vi "2.0 EMGtoOMG OFFLINE functional keyboard.vi"() -> ()   [LabVIEW 2018]
panel:
  out "charSearch":dbl[](array[numeric])
  in  "Sig 3":bool
  in  "Sig 2":bool
  in  "Sig 1":bool
  out "return value":string
  out "Array":string[](array[string])
  out "c":i32[](array[numeric])
  out "state":dbl[](array[numeric])
  out "charSearch":dbl[](array[numeric])
  out "seq70-104":dbl[](array[numeric])
  out "seq00-34":dbl[](array[numeric])
  out "setID":dbl[](array[numeric])
  out "seq35-69":dbl[](array[numeric])
  in  "Amplitude 3":dbl=1.0 caption="Amplitude"
  in  "Amplitude 2":dbl=1.0 caption="Amplitude"
  in  "Amplitude":dbl=1.0
  in  "stop":bool
  in  "module path":path
  # "1-1-1 -> invalid\n\n1-1-2 -> Set 1 ' abcdeABCDE'\n\n1-1-3 -> Set 2 ' fghijkFGHIJK' \n\n1-2-1 -> Set 3 ' lmnopLMNOP' \n\n1-2-2 -> Set 4 ' qrstuQRSTU'\n\n1-2-3 -> Set 5 ' vwxyzVWXYZ' \n\n1-3-1 -> Set 6 ' .,!>\\'\\\"@#&_-+=' \n\n1-3-2 -> Set 7 ' ()[]<>/\\|%^*~'\n\n1-3-3 -> Set 8 ' 0123456789'"
  # "To the right of the three signals is a \"state\" indicator. \n\nState 1 - \"Unknown\" \n-Program is  waiting for a 1 to start building setID.\n-While in State 1, 2s and 3s don't do anything. \n- Enter a 1 to change to State 2 and begin recording a setID.\n\nState 2 - \"Find\"\n-Program stores next two inputs into setID.\n-The ID can be seen in the setID indicator. The first the numbers is the ID of the set, the 4th number is the associated number of the set (1-8)\n-An ID of 1-1-1 is invalid, and this will change the state back to state 1. \n-All other sets are valid and change state to State 3\n\nState 3 - \"Nav\"\n-Program cycles through and selects a chosen character in a set\n-Repeating 3s will cycle forward through a set, currently selected character is in {}\n-2 will enter the selected character and stay in the current set, and reset the cycle\n-1 will enter the selected character and acts as the first digit in a new setID, and changes to State 2\n\nUse the following sequence as practice:\n2332-121-3-113-3333-122-33333333333-3333-1\n\n2332 does nothing\n121 chooses Set 3\n3 cycles through Set 3\n113 selects character and chooses Set 2\n3333 cycles through Set 2\n122 selects character and chooses Set 4\n33333333333 (eleven 3s) cycles completely through Set 4\n3333 cycles through set 4\n1 selects character"
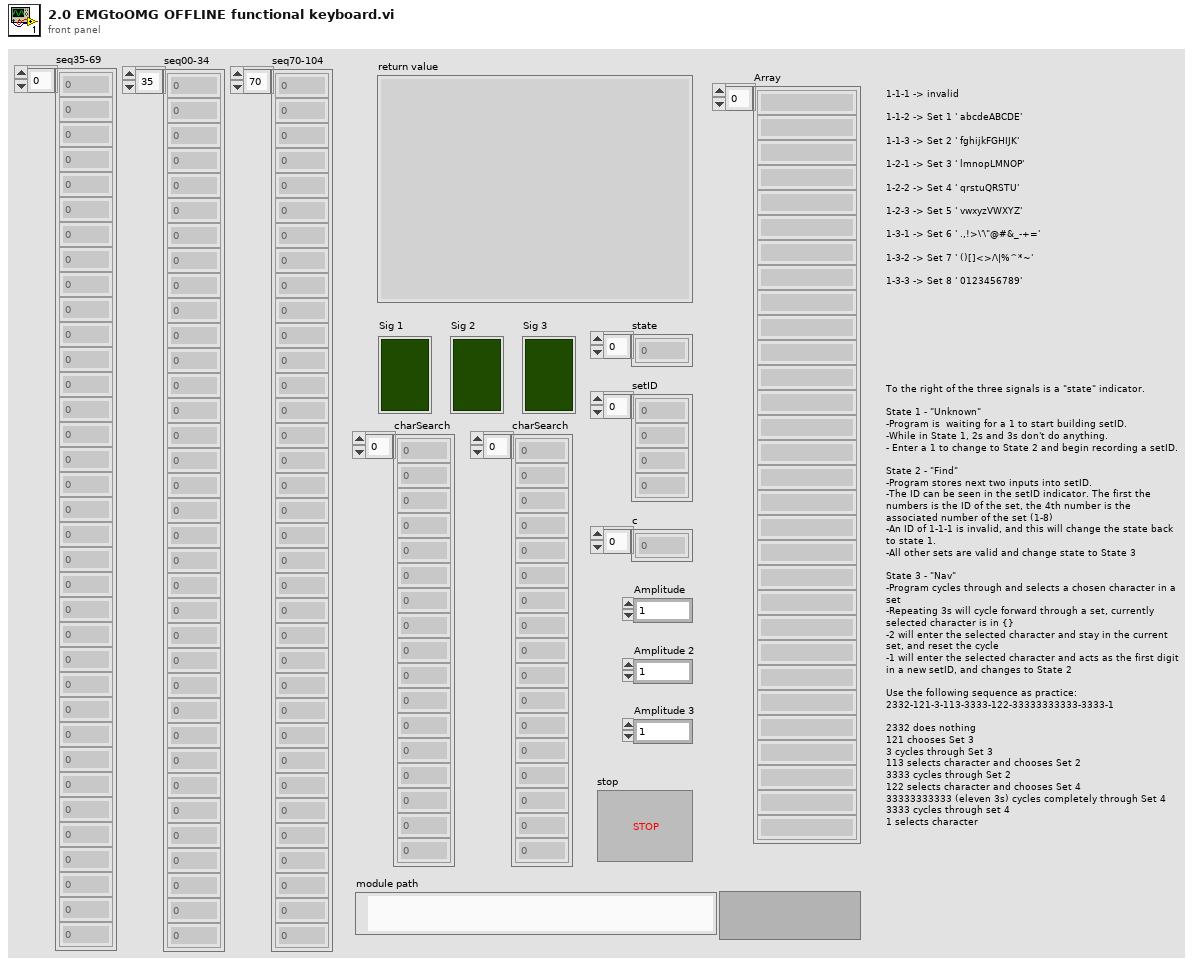
[diagram p1: front panel]
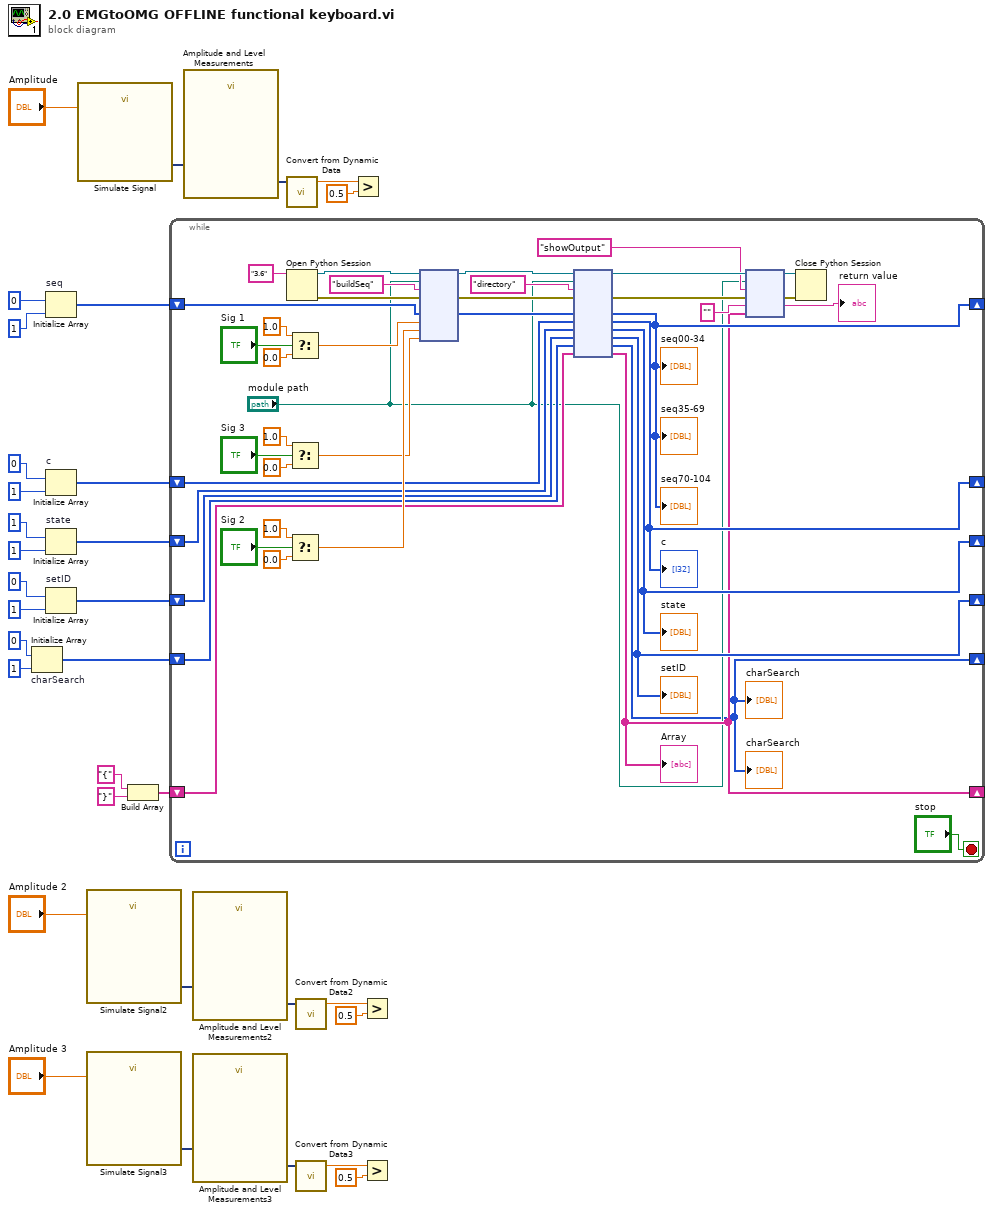
[diagram p0: block diagram]
diagram:
  n1 = Initialize Array "charSearch"(0, 1 ("dimension size")) -> (w28:i32[])
  n2 = Initialize Array "seq"(0, 1 ("dimension size")) -> (w33:i32[])
  n3 = Initialize Array "c"(0, 1 ("dimension size")) -> (w26:i32[])
  n4 = Initialize Array "state"(1, 1 ("dimension size")) -> (w23:i32[])
  n5 = Initialize Array "setID"(0, 1 ("dimension size")) -> (w29:i32[])
  n6 = call "Simulate Signal"("Amplitude"="Amplitude") -> ("Sine"=w7:dynamicdata)  [unwired: 13 in, 1 out]
  n7 = call "Simulate Signal2"("Amplitude"="Amplitude 2") -> ("Sine"=w17:dynamicdata)  [unwired: 13 in, 1 out]
  n8 = call "Simulate Signal3"("Amplitude"="Amplitude 3") -> ("Sine"=w12:dynamicdata)  [unwired: 13 in, 1 out]
  n9 = Build Array("{", "}") -> (w20:string[])
  n10 = while {
    shift-right: [w55] -> _
    shift-left: w33 -> [w66]
    shift-right: [w51] -> _
    shift-left: w29 -> [w54]
    shift-right: [w34] -> _
    shift-left: w28 -> [w53]
    shift-right: [w44] -> _
    shift-left: w20 -> [w52]
    shift-right: [w49] -> _
    shift-left: w23 -> [w50]
    shift-right: [w47] -> _
    shift-left: w26 -> [w48]
    stop <- "stop" stop-if-true
    n11 = Open Python Session(python version="3.6" ("Python version")) -> (session out=w73:refnum<k35>, error out=w72:errorcluster)  [unwired: 2 in]
    n12 = Select(t=1.0, s="Sig 1", f=0.0) -> (s? t:f=w69:dbl)
    n13 = Select(t=1.0, s="Sig 3", f=0.0) -> (s? t:f=w60:dbl)
    n14 = Select(t=1.0, s="Sig 2", f=0.0) -> (s? t:f=w61:dbl)
    n15 = node(w73, "module path", "buildSeq" ("function name"), w72, w66, w69, w61, w60) -> (w59:refnum<k35>, w58:errorcluster, w56:i32[])  [unwired: 5 in, 2 out]
    n16 = node(w59, "module path", "directory" ("function name"), w58, w56, w48, w50, w54, w53, w52) -> (w43:refnum<k35>, w41:errorcluster, w55:i32[], w47:i32[], w49:i32[], w51:i32[], w34:i32[], w44:string[])  [unwired: 2 in, 2 out]
    "seq35-69" <- w55
    "setID" <- w51
    "seq00-34" <- w55
    "seq70-104" <- w55
    "charSearch" <- w34
    "state" <- w49
    "c" <- w47
    "Array" <- w44
    "charSearch" <- w34
    n17 = node(w43, "module path", "showOutput" ("function name"), w41, "", w44) -> (w42:refnum<k35>, w40:errorcluster, →"return value":string)  [unwired: 1 in, 2 out]
    n18 = Close Python Session(session in=w42, error in=w40) -> ()  [unwired: 1 out]
  }
  n19 = call "Amplitude and Level Measurements"("Signals"=w7) -> ("RMS"=w8:dynamicdata)  [unwired: 13 in, 1 out]
  n20 = call "Amplitude and Level Measurements2"("Signals"=w17) -> ("RMS"=w18:dynamicdata)  [unwired: 13 in, 1 out]
  n21 = call "Amplitude and Level Measurements3"("Signals"=w12) -> ("RMS"=w13:dynamicdata)  [unwired: 13 in, 1 out]
  n22 = call "Convert from Dynamic Data"("Dynamic Data Type"=w8) -> ("Scalar"=w9:dbl)  [unwired: 3 in]
  n23 = call "Convert from Dynamic Data2"("Dynamic Data Type"=w18) -> ("Scalar"=w19:dbl)  [unwired: 3 in]
  n24 = call "Convert from Dynamic Data3"("Dynamic Data Type"=w13) -> ("Scalar"=w14:dbl)  [unwired: 3 in]
  n25 = Greater?(x=w9, y=0.5) -> ()  [unwired: 1 out]
  n26 = Greater?(x=w19, y=0.5) -> ()  [unwired: 1 out]
  n27 = Greater?(x=w14, y=0.5) -> ()  [unwired: 1 out]
